vi "Obstacle Avoidance Loop.vi"   [LabVIEW 2009]
uses:
  <vilib>/Platform/TimedLoop/XDataNode/XDataNode.xnode
  <vilib>/Platform/TimedLoop/XDataNode/loadlvalarms.vi
  <vilib>/Platform/TimedLoop/XDataNode/timing_clust.ctl
  <vilib>/Platform/TimedLoop/XDataNode/nitl_modes.ctl
  <vilib>/Platform/TimedLoop/XDataNode/wakeup.ctl
  Functional Global Variables/Actions for FG's.ctl
  <vilib>/Platform/TimedLoop/XDataNode/XDNodeRunTimeDep.lvlib
types:
  T1 = typedef "XDNodeRunTimeDep.lvlib/timing_clust.ctl" = cluster{"Expected End [f-1]":u64, "Actual End [f-1]":u64, "Finished Late? [f-1]":bool, "Expected End [i-1]":u64, "Actual End [i-1]":u64, "Finished Late? [i-1]":bool, "Expected Start [i]":u64, "Actual Start [i]":u64, "Expected Start [f]":u64, "Actual Start [f]":u64, "Source Name":string, "Structure Name":string, "Period":i64, "Deadline":i64, "Offset":i64, "Start":i64, "Priority":i32, "Timeout":i32, "Mode":T2, "Wakeup Reason":T3, "Error":errorcluster, "Source Type":string, "Secondary Source Type":string, "Global End Time":u64, "Global Start Time":u64, "Frame Duration":u64, "Iteration Duration":u64, "Assigned CPU":i32, "I/O Scan Engine Mode":u32}
  T2 = typedef "XDNodeRunTimeDep.lvlib/nitl_modes.ctl" = enum32{"No Change", "Process missed periods, maintain original phase", "Discard missed periods, maintain original phase", "Process missed periods, ignore original phase", "Discard missed periods, ignore original phase"}
  T3 = typedef "XDNodeRunTimeDep.lvlib/wakeup.ctl" = enum32{"Normal", "Aborted", "Asynchronous wakeup", "Timing source error", "Timed loop error", "Timeout"}
  T4 = typedef "Actions for FG's.ctl" = enum16{"Read", "Write"}
  T5 = typedef "SICK Array.ctl" = u16[]
  T6 = typedef "Motor Command.ctl" = cluster{"Speed":i16, "Turn":i16}
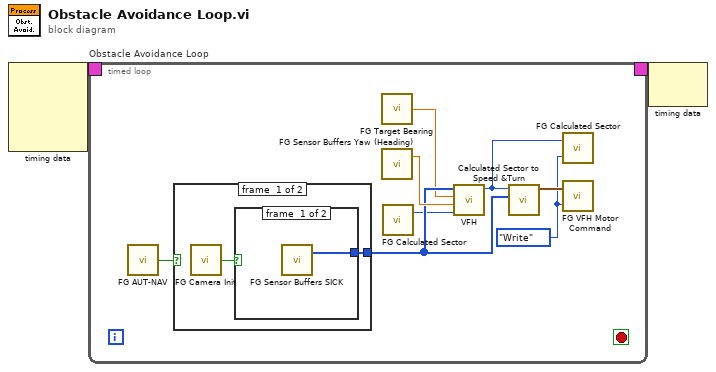
[diagram p0: block diagram]
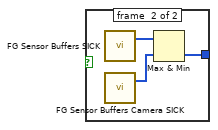
[diagram p2: hidden frame]
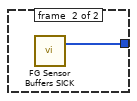
[diagram p3: hidden frame]
diagram:
  n1 = node-c288() -> (w2:T1)  [unwired: 4 in]
  n2 = timed-loop "Obstacle Avoidance Loop" {
    timing: w2 -> [_]
    timing-out: [_] -> w1
    stop <- _ stop-if-true
    w3 = Actions_for_FG's."Write" ("FG Action")
    n3 = call "FG AUT-NAV.vi"() -> ("Aut/!Nav out"=w4:bool)  [unwired: 2 in]
    n4 = case shown="True" w4 {
      tunnel: [w12 w17] -> w8
      frame #0 {
        n5 = call "FG Camera Init.vi"() -> ("Camera Init out"=w11:bool)  [unwired: 2 in]
        n6 = case shown="True" w11 {
          tunnel: [w13 w15] -> w12
          frame #0 {
            n7 = call "FG Sensor Buffers SICK.vi"() -> ("SICK Buffer out"=w13:T5)  [unwired: 3 in]
          }
          frame #1 {
            n8 = call "FG Sensor Buffers SICK.vi"() -> ("SICK Buffer out"=w16:T5)  [unwired: 3 in]
            n9 = call "FG Sensor Buffers Camera SICK.vi"() -> ("Camera SICK Buffer out"=w14:T5)  [unwired: 3 in]
            n10 = Max & Min(x=w16, y=w14) -> (min(x,y)=w15:T5)  [unwired: 1 out]
          }
        }
      }
      frame #1 {
        n11 = call "FG Sensor Buffers SICK.vi"() -> ("SICK Buffer out"=w17:T5)  [unwired: 3 in]
      }
    }
    n12 = call "FG Target Bearing.vi"() -> ("Target Bearing out"=w7:dbl)  [unwired: 2 in]
    n13 = call "FG Sensor Buffers Yaw (Heading).vi"() -> ("Yaw Buffer Out"=w9:dbl)  [unwired: 3 in]
    n14 = call "FG Calculated Sector.vi"() -> ("Target sector out"=w5:i16)  [unwired: 3 in]
    n15 = call "VFH.vi"("Previous Calculated Sector"=w5, "Compass Bearing (degrees)"=w9, "Target Bearing (degrees)"=w7, "RAW SICK Data"=w8) -> ("Calculated sector"=w6:i16)  [unwired: 7 in]
    n16 = call "Calculated Sector to Speed &Turn.vi"("RAW SICK Data"=w8, "Calculated Sector"=w6) -> ("Motor Commands"=w10:T6)  [unwired: 9 in]
    n17 = call "FG Calculated Sector.vi"("FG Action (Read)"=w3, "Target sector in"=w6) -> ()  [unwired: 1 in, 1 out]
    n18 = call "FG VFH Motor Command.vi"("FG Action"=w3, "Motor Command in"=w10) -> ()  [unwired: 1 in, 1 out]
  }
  n19 = node-c288(w1) -> ()  [unwired: 1 out]
